vi "Read DMM.vi"(8 "error in (no error)":errorcluster, 11 "IVI Refnum in":refnum<k15>) -> (3 "Measurement":dbl)   [LabVIEW 2021, in "DMM 20.lvlib"]
uses:
  DMM 20.lvlib
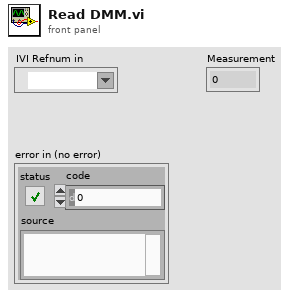
[diagram p1: front panel]
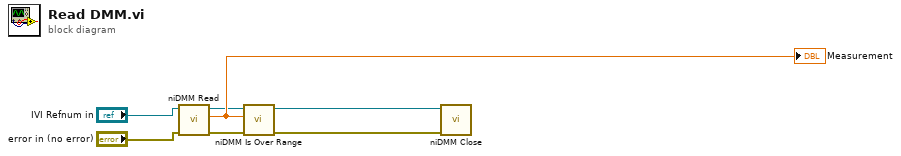
[diagram p0: block diagram]
diagram:
  n1 = call <instrlib>:"niDMM Read.vi"("error in (no error)"="error in (no error)", "instrument handle"="IVI Refnum in") -> ("error out"=w4:errorcluster, "Measurement"=w5:dbl, "instrument handle out"=w3:refnum<k15>)  [unwired: 7 in]
  "Measurement" <- w5
  n2 = call <instrlib>:"niDMM Is Over Range.vi"("error in (no error)"=w4, "Measurement"=w5, "instrument handle"=w3) -> ("error out"=w7:errorcluster, "instrument handle out"=w6:refnum<k15>)  [unwired: 6 in, 1 out]
  n3 = call <instrlib>:"niDMM Close.vi"("error in (no error)"=w7, "instrument handle"=w6) -> ()  [unwired: 9 in, 1 out]
